vi "Start Counter.vi"(1 "Counter":tag="Dev2/ctr0", 2 "Device":tag="Dev2") -> (0 "Error":errorcluster)   [LabVIEW 2011]
uses:
  <vilib>/DAQmx/create/channels.llb/DAQmx Create Channel (CI-Count Edges).vi
panel:
  # "by Paul Nathan, 01/03/2012"
  # "Revisions:\nDate       Desc.      Auth.\nx               x               x"
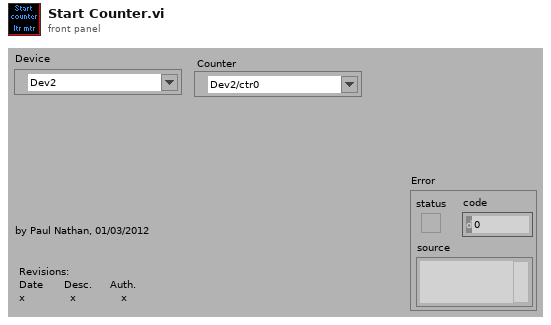
[diagram p1: front panel]
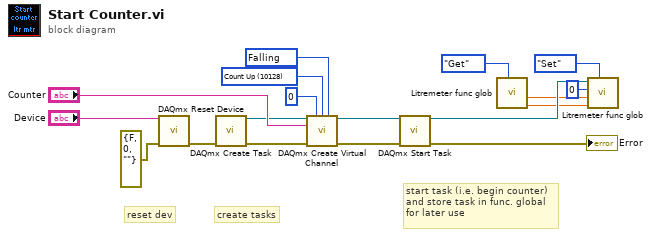
[diagram p0: block diagram]
diagram:
  w8 = 10171 items=["Rising"=10280, "Falling"=10171] ("edge")
  w9 = 10128 items=["Count Up"=10128, "Count Down"=10124, "Externally Controlled"=10326] ("count direction")
  # "start task (i.e. begin counter) and store task in func. global for later use"
  # "create tasks"
  # "reset dev"
  n1 = call <vilib>:"DAQmx Reset Device.vi"("device in"="Device", "error in"=errorcluster {"status"=FALSE, "code"=0, "source"=""}) -> ("error out"=w14:errorcluster)  [unwired: 13 in]
  n2 = call <vilib>:"DAQmx Create Task.vi"("error in"=w14) -> ("task out"=w11:refnum<k21>, "error out"=w12:errorcluster)  [unwired: 13 in]
  n3 = call-poly <vilib>:"DAQmx Create Virtual Channel.vi"("task in"=w11, "initial count"=u32 0, "count direction"=w9, "edge"=w8, "counter"="Counter", "error in"=w12) -> ("task out"=w15:refnum<k21>, "error out"=w16:errorcluster)  [unwired: 8 in]
  n4 = call <vilib>:"DAQmx Start Task.vi"("task/channels in"=w15, "error in"=w16) -> ("task out"=w5:refnum<k21>, "error out"=→"Error":errorcluster)  [unwired: 12 in]
  n5 = call "Litremeter func glob.vi"("Action"=enum16{"Get", "Set"}."Get") -> ("Offset Litres out"=w2:dbl, "Litres / pulse out"=w1:dbl)  [unwired: 4 in, 3 out]
  n6 = call "Litremeter func glob.vi"("Action"=enum16{"Get", "Set"}."Set", "Offset Litres in"=w2, "Litres / pulse in"=w1, "Pulse count in"=u32 0, "Counter task in"=w5) -> ()  [unwired: 5 out]
